vi "GSP_F2_Global.vi"() -> ()   [LabVIEW 2015]
uses:
  SystemUtil/MotorStates.ctl
  SystemUtil/ThreadStates.ctl
panel:
  in  "F2_Name":string
  in  "F2 Thread State":T1
  in  "F2 Motor State":T2
  in  "F2 CPU Temp":dbl
  out "F2 Online":bool
  in  "Filter#":i32
  in  "Offset to 1st Pos":i32
  in  "Counts per Position":dbl=6222.17 format="%.2f"
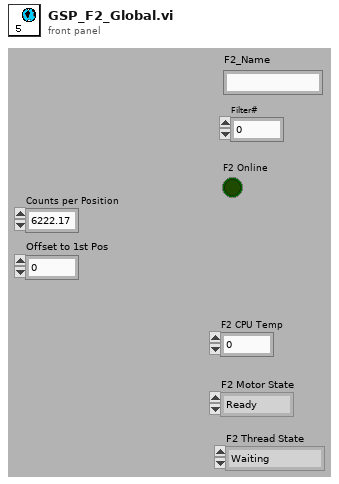
[diagram p1: front panel]
types:
  T1 = typedef "ThreadStates.ctl" = enum16{"Waiting", "Scripting", "Uninitialized", "Error"}
  T2 = typedef "MotorStates.ctl" = enum16{"Ready", "Moving", "Uninitialized", "Error"}
diagram:
